vi "Deploy Firmware.vi"() -> ()   [LabVIEW 2011, in "LVH-LINX.lvlib"]
uses:
  LVH-LINX.lvlib
  Type Defs/Device Family.ctl
  Type Defs/Deploy Firmware State.ctl
panel:
  in  "Device Family Enum":T1
  out "Error Out":errorcluster
  in  "Error In":errorcluster
  out "Tab Control":T2(tab)
  in  "Device Help":bool
  in  "Firmware Program Interface":u16(ring) items=["Serial / USB"]
  in  "Device Type":u16(ring) items=["chipKIT Uno32", "chipKIT uC32", "chipKIT Max32", "chipKIT DP32"]
  in  "Device Family":u16(ring) items=["National Instruments", "Digilent", "Arduino"]
  in  "Device Cancel":bool
  in  "Device Next":bool
  in  "Int Help":bool
  in  "Int Previous":bool
  in  "Int Cancel":bool
  in  "Int Next":bool
  out "Interface Config":enum32{"N/A", "Serial / USB", "USB", "TCP"}(tab)
  in  "COM Port":refnum<visa-resource-name>
  in  "FWV Help":bool
  in  "FWV Cancel":bool
  in  "FWV Next":bool
  in  "FWV Previous":bool
  in  "Firmware Version":u16(ring)
  in  "Summary Next":bool
  in  "Summary Help":bool
  # "Choose The Device"
  # "!!! Could Add Test Connection Button Here !!!"
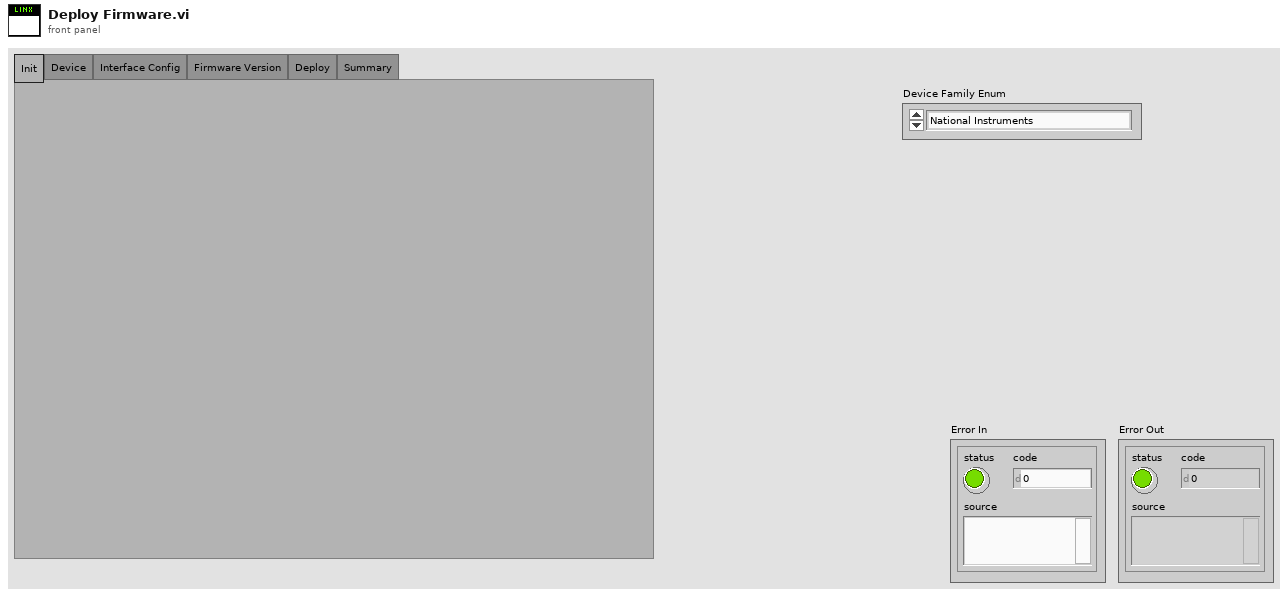
[diagram p1: front panel]
types:
  T1 = typedef "LVH-LINX.lvlib/Device Family.ctl" = enum8{"National Instruments", "Digilent", "Arduino"}
  T2 = enum32{"Init", "Device", "Interface Config", "Firmware Version", "Deploy", "Summary"}
  T3 = typedef "LVH-LINX.lvlib/Deploy Firmware State.ctl" = enum32{"Init", "Device", "Interface Config", "Firmware Version", "Deploy", "Summary"}
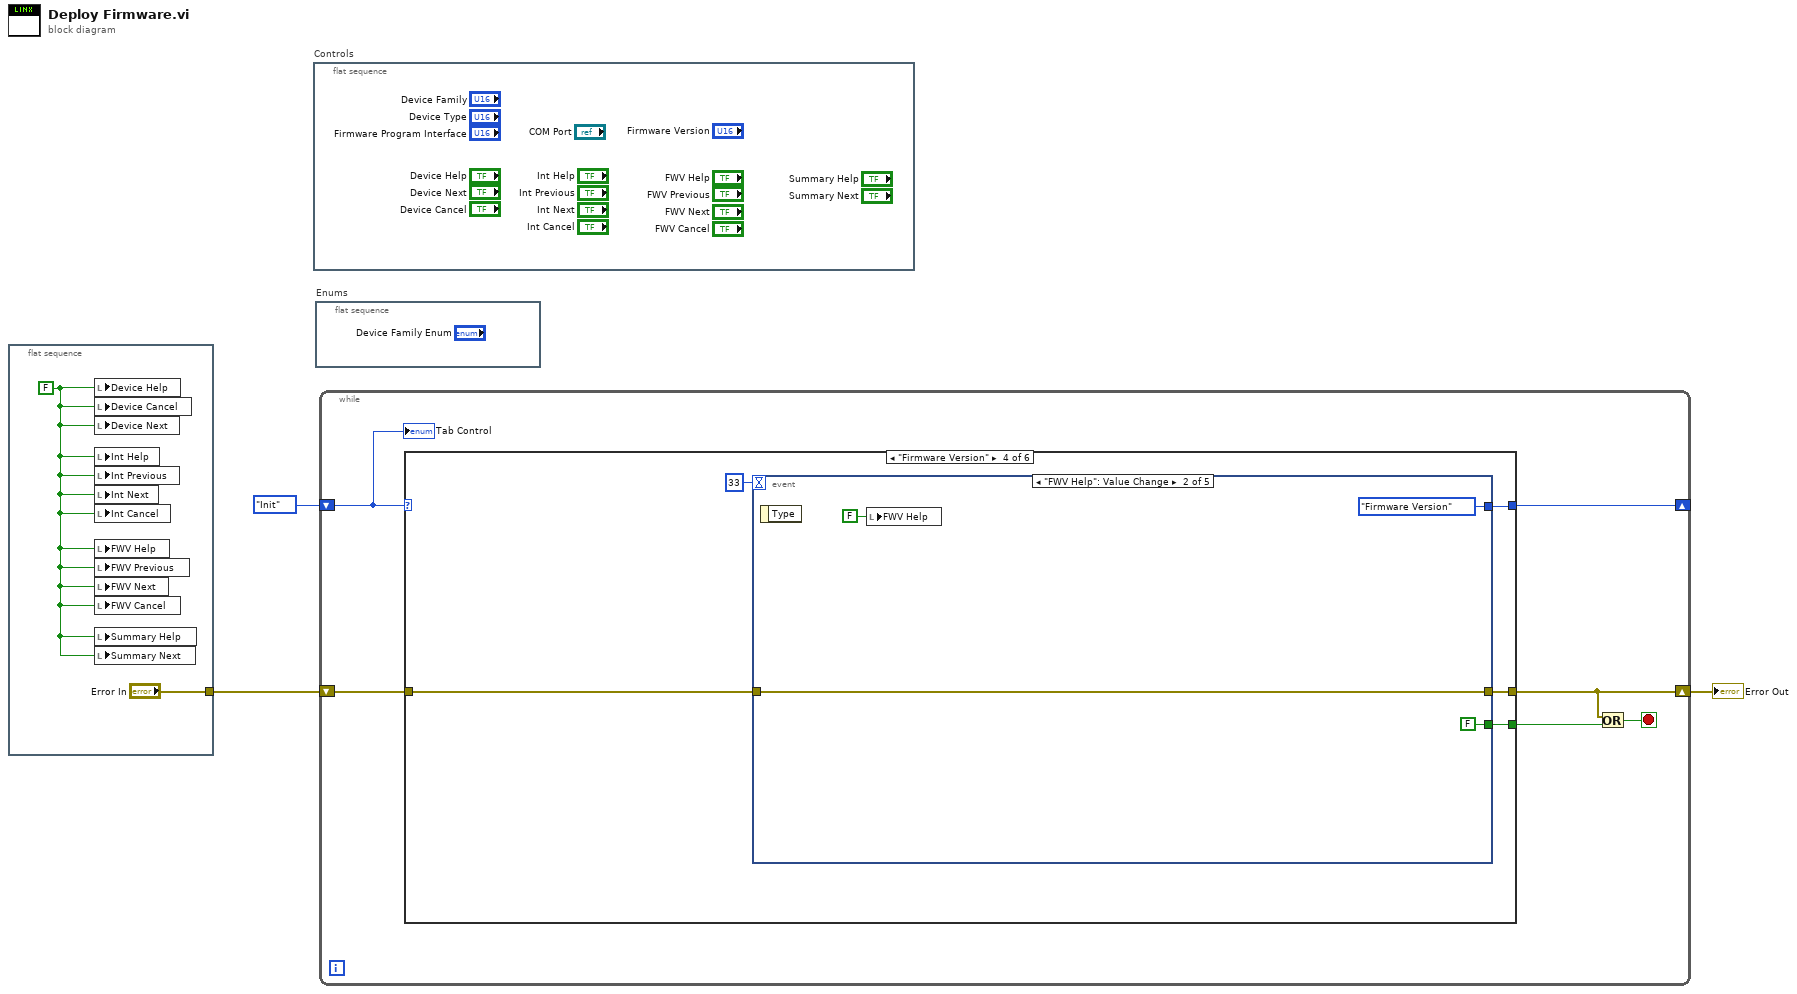
[diagram p0: block diagram]
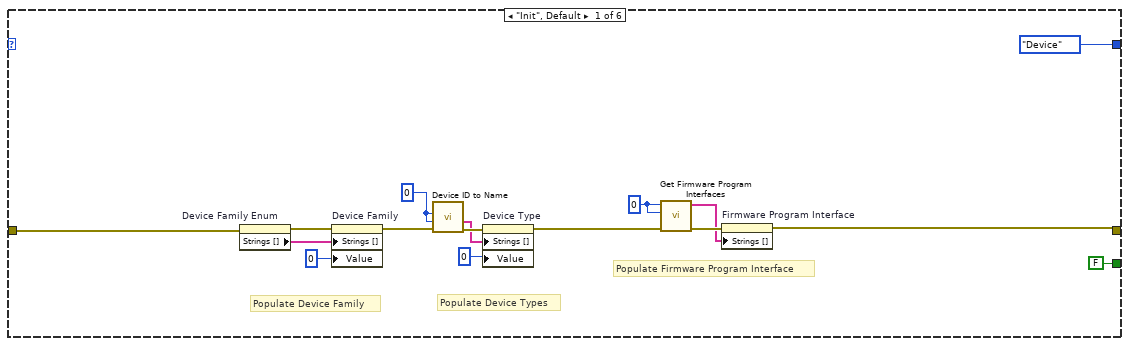
[diagram p2: hidden frame]
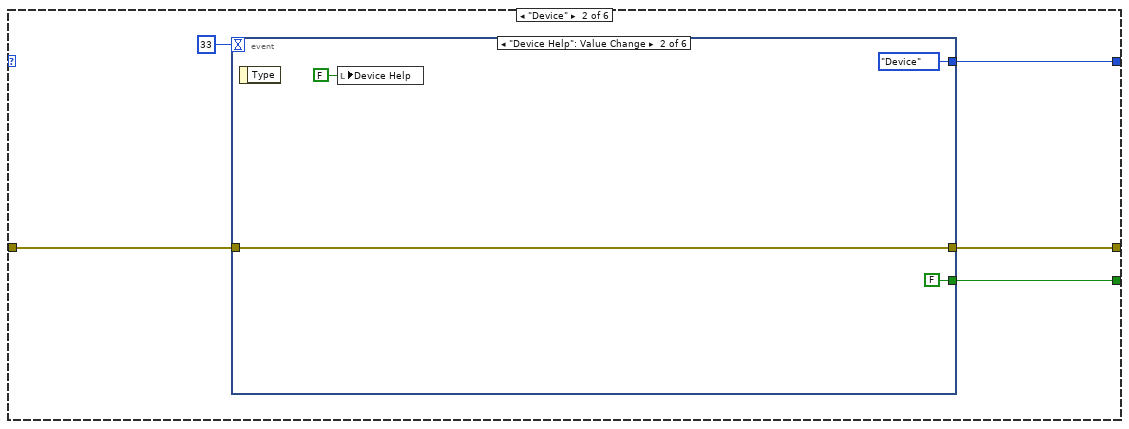
[diagram p3: hidden frame]
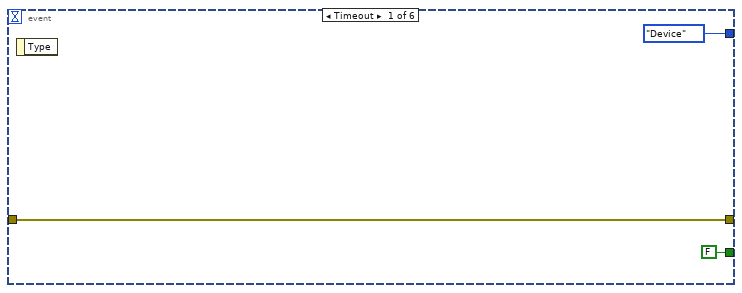
[diagram p4: hidden frame]
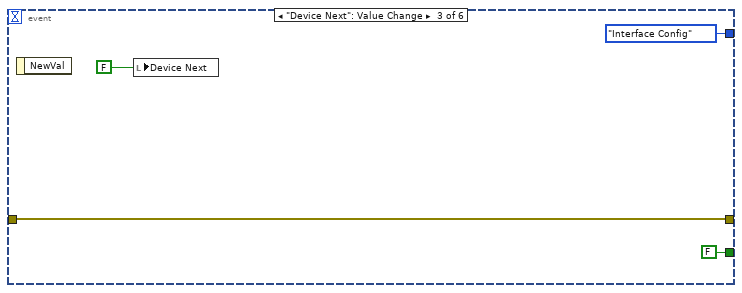
[diagram p5: hidden frame]
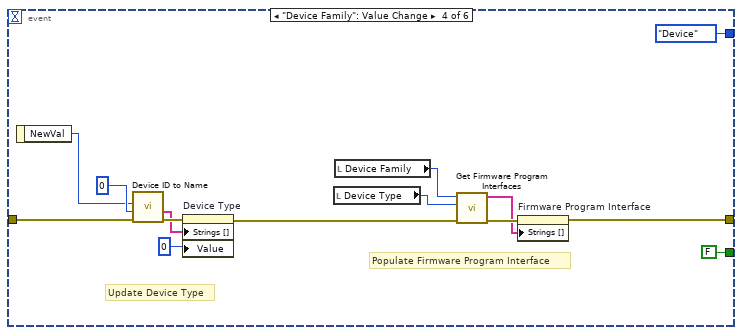
[diagram p6: hidden frame]
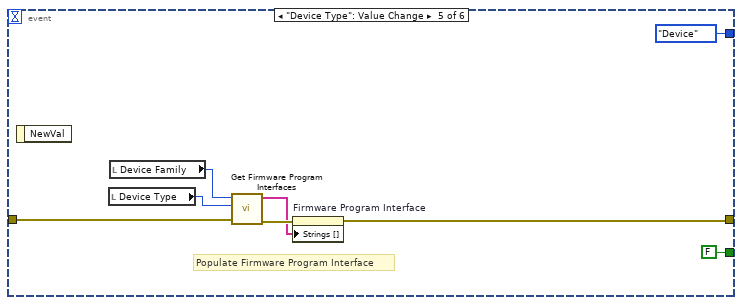
[diagram p7: hidden frame]
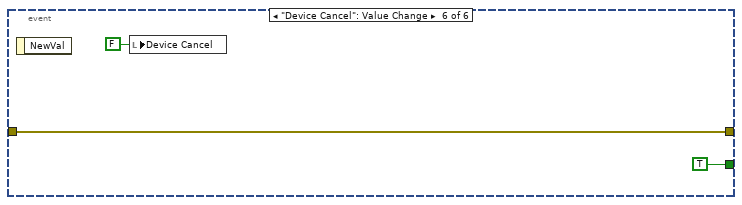
[diagram p8: hidden frame]
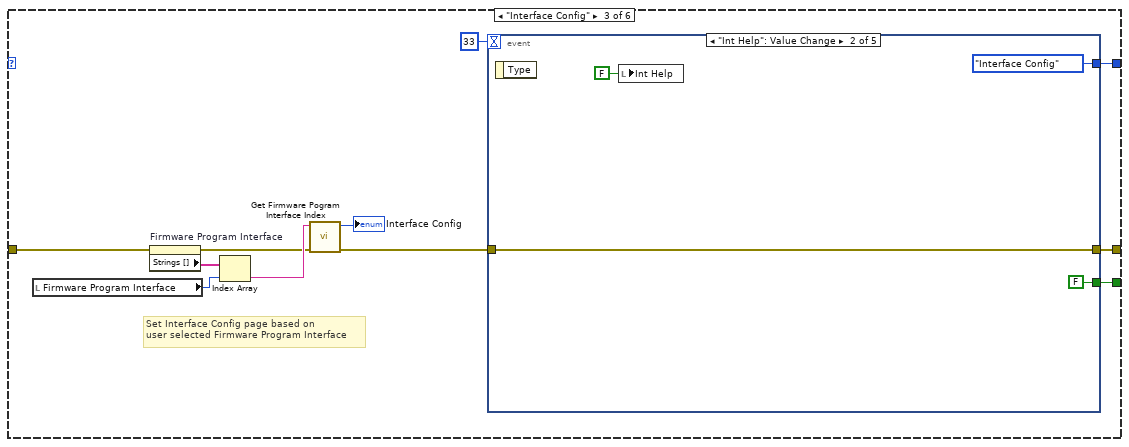
[diagram p9: hidden frame]
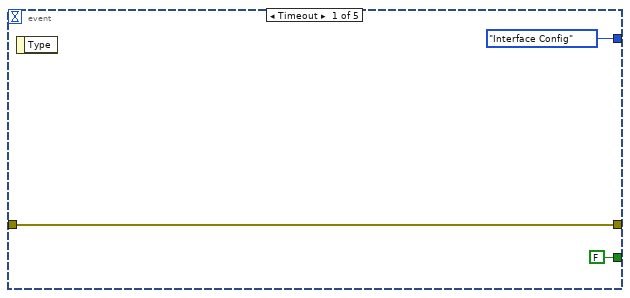
[diagram p10: hidden frame]
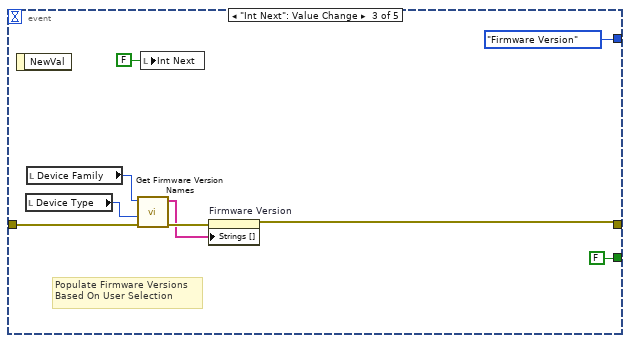
[diagram p11: hidden frame]
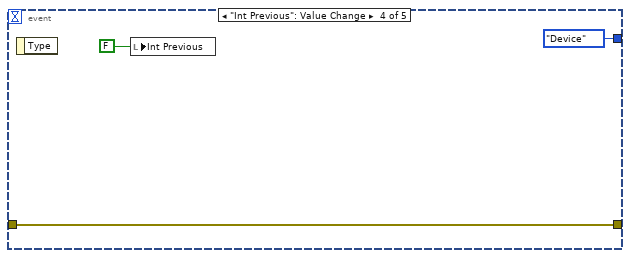
[diagram p12: hidden frame]
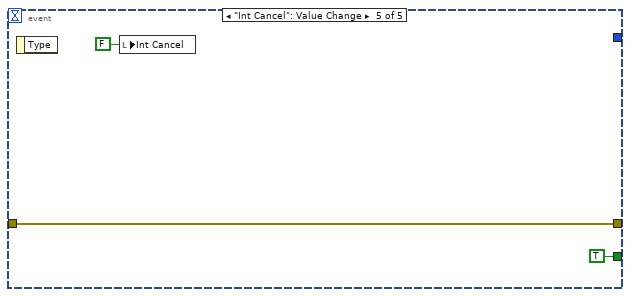
[diagram p13: hidden frame]
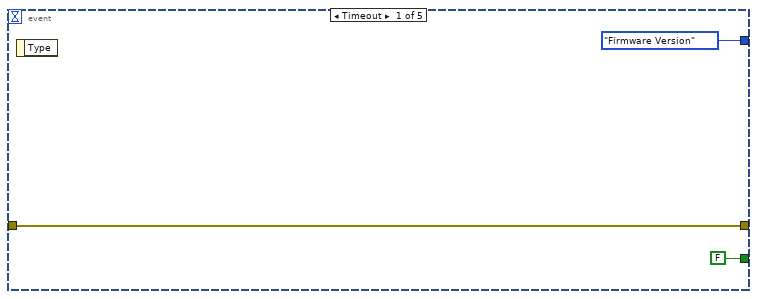
[diagram p14: hidden frame]
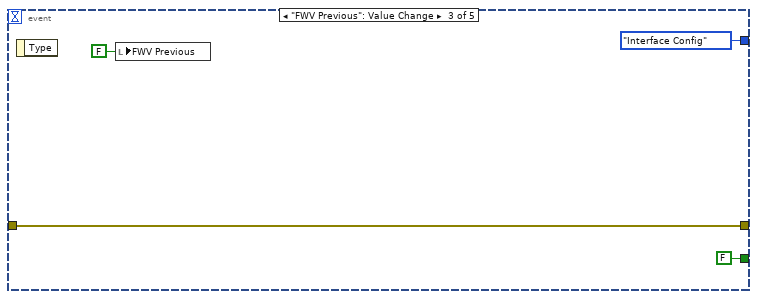
[diagram p15: hidden frame]
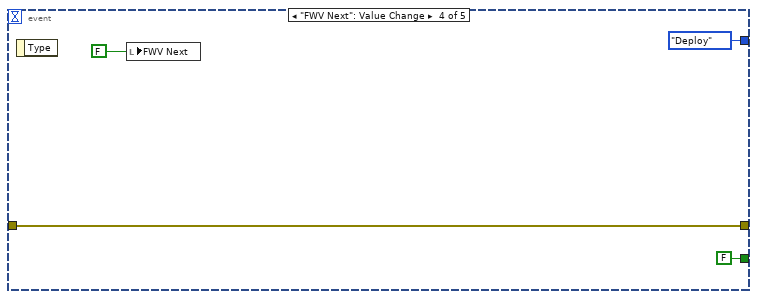
[diagram p16: hidden frame]
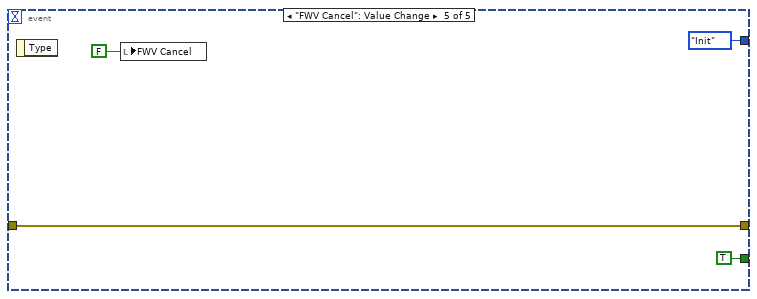
[diagram p17: hidden frame]
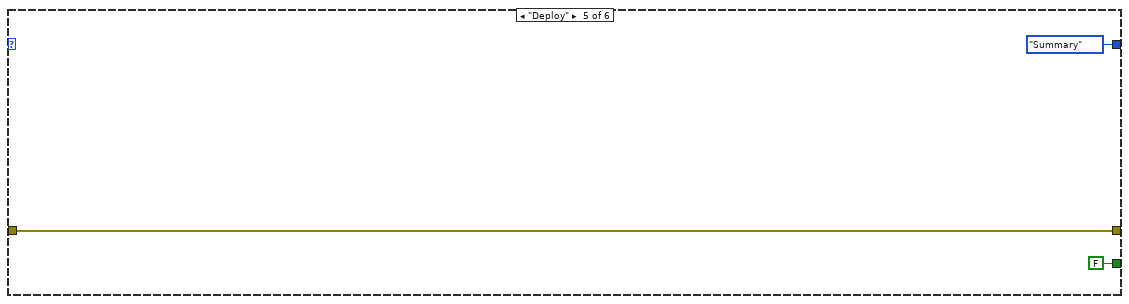
[diagram p18: hidden frame]
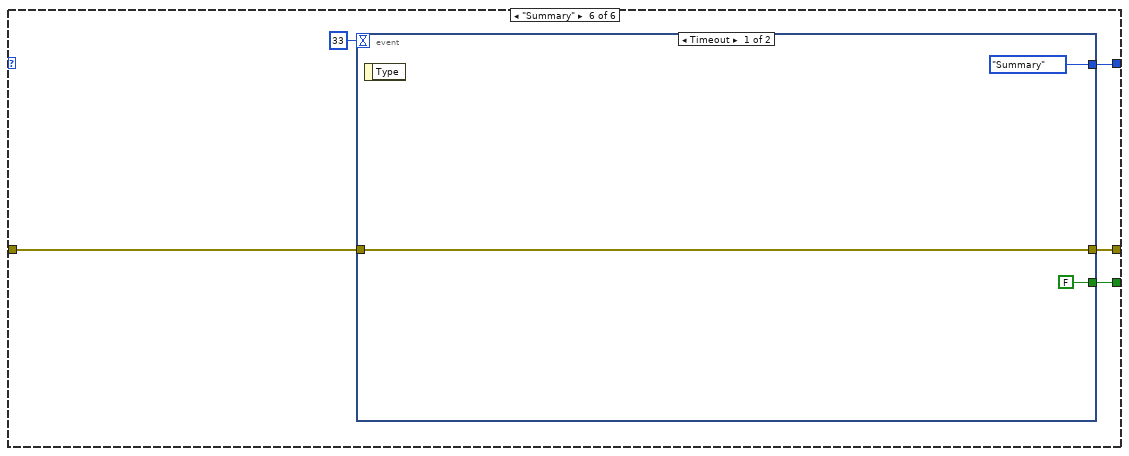
[diagram p19: hidden frame]
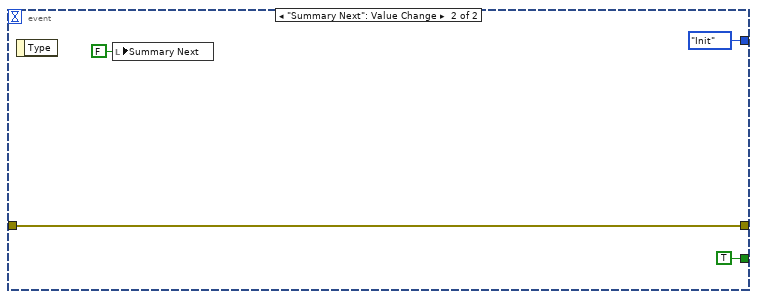
[diagram p20: hidden frame]
diagram:
  n1 = flat-sequence {
    tunnel: ["Error In"] -> w1
    frame #0 {
      w4 = FALSE ("Cancel")
      n2 = local write "Device Help"(w4) -> ()
      n3 = local write "Device Cancel"(w4) -> ()
      n4 = local write "Device Next"(w4) -> ()
      n5 = local write "Int Help"(w4) -> ()
      n6 = local write "Int Previous"(w4) -> ()
      n7 = local write "Int Next"(w4) -> ()
      n8 = local write "Int Cancel"(w4) -> ()
      n9 = local write "FWV Help"(w4) -> ()
      n10 = local write "FWV Previous"(w4) -> ()
      n11 = local write "FWV Next"(w4) -> ()
      n12 = local write "FWV Cancel"(w4) -> ()
      n13 = local write "Summary Help"(w4) -> ()
      n14 = local write "Summary Next"(w4) -> ()
    }
  }
  n15 = flat-sequence "Controls" {
    frame #0 {
    }
  }
  n16 = flat-sequence "Enums" {
    frame #0 {
    }
  }
  n17 = while {
    shift-right: [w9] -> _
    shift-left: Deploy_Firmware_State."Init" ("Deploy Firmware State") -> [w11]
    shift-right: [w8] -> w2
    shift-left: w1 -> [w10]
    stop <- w7 stop-if-true
    n18 = case shown="\"Firmware Version\"" w11 {
      tunnel: [w14 w31 w72 w106 w128 w133] -> w8
      tunnel: w10 -> [w13 w30 w78 w105 w128 w132]
      tunnel: [Deploy_Firmware_State."Device" ("Deploy Firmware State") w29 w79 w103 Deploy_Firmware_State."Summary" ("Deploy Firmware State") w130] -> w9
      tunnel: [FALSE w28 w69 w102 FALSE w129] -> w6
      frame "Init", Default {
        w15 = u32 0 ("Device Family")
        w21 = u32 0 ("Device Family")
        # "Populate Firmware Program Interface"
        # "Populate Device Types"
        # "Populate Device Family"
        n19 = property on="Device Family Enum" class="Enum (strict)"(error in=w13) -> (error out=w26:errorcluster, "Strings []"=w25:string[])  [unwired: 1 in, 1 out]
        n20 = property on="Device Family" class="Ring (strict)"(error in=w26, "Strings []"=w25, "Value"=u16 0 ("Device Family")) -> (error out=w23:errorcluster)  [unwired: 1 in, 1 out]
        n21 = call "Device ID to Name.vi"("Error In"=w23, "Device ID"=w21, "Device Family"=w21) -> ("Error Out"=w22:errorcluster, "Devices In Family"=w20:string[])  [unwired: 5 in, 2 out]
        n22 = property on="Device Type" class="Ring (strict)"(error in=w22, "Strings []"=w20, "Value"=u16 0 ("Device Family")) -> (error out=w16:errorcluster)  [unwired: 1 in, 1 out]
        n23 = call "Get Firmware Program Interfaces.vi"("Error In"=w16, "Device ID"=w15, "Device Family"=w15) -> ("Error Out"=w18:errorcluster, "Firmware Program Interfaces"=w17:string[])  [unwired: 7 in]
        n24 = property on="Firmware Program Interface" class="Ring (strict)"(error in=w18, "Strings []"=w17) -> (error out=w14:errorcluster)  [unwired: 1 in, 1 out]
      }
      frame "Device" {
        n25 = event shown="[1] \"Device Help\": Value Change" {
          selector: _ -> [_ _ _ _ _ _]
          dyn-events: _ -> [_ _ _ _ _ _]
          timeout: 33 -> [_ _ _ _ _ _]
          tunnel: [w35 w37 w42 w46 w62 w67] -> w31
          tunnel: w30 -> [w35 w37 w42 w53 w65 w67]
          tunnel: [Deploy_Firmware_State."Device" ("Deploy Firmware State") Deploy_Firmware_State."Device" ("Deploy Firmware State") Deploy_Firmware_State."Interface Config" ("Deploy Firmware State") Deploy_Firmware_State."Device" ("Deploy Firmware State") Deploy_Firmware_State."Device" ("Deploy Firmware State") _] -> w29
          tunnel: [FALSE FALSE FALSE FALSE FALSE TRUE] -> w28
          event Timeout {
            n26 = event-data() -> ()  [unwired: 1 in, 1 out]
          }
          event "Device Help": Value Change {
            n27 = event-data() -> ()  [unwired: 1 in, 1 out]
            n28 = local write "Device Help"(FALSE ("Device Help")) -> ()
          }
          event "Device Next": Value Change {
            n29 = event-data() -> ()  [unwired: 1 in, 1 out]
            n30 = local write "Device Next"(FALSE ("Next")) -> ()
          }
          event "Device Family": Value Change {
            # "Populate Firmware Program Interface"
            # "Update Device Type"
            n31 = event-data() -> ("NewVal"=w52:u16)  [unwired: 1 in]
            n32 = call "Device ID to Name.vi"("Error In"=w53, "Device ID"=u32 0 ("Device Family"), "Device Family"=w52) -> ("Error Out"=w57:errorcluster, "Devices In Family"=w55:string[])  [unwired: 5 in, 2 out]
            n33 = property on="Device Type" class="Ring (strict)"(error in=w57, "Strings []"=w55, "Value"=u16 0 ("Device Family")) -> (error out=w45:errorcluster)  [unwired: 1 in, 1 out]
            n34 = local read "Device Type"() -> (w48:u16)
            n35 = local read "Device Family"() -> (w47:u16)
            n36 = call "Get Firmware Program Interfaces.vi"("Error In"=w45, "Device ID"=w48, "Device Family"=w47) -> ("Error Out"=w50:errorcluster, "Firmware Program Interfaces"=w49:string[])  [unwired: 7 in]
            n37 = property on="Firmware Program Interface" class="Ring (strict)"(error in=w50, "Strings []"=w49) -> (error out=w46:errorcluster)  [unwired: 1 in, 1 out]
          }
          event "Device Type": Value Change {
            # "Populate Firmware Program Interface"
            n38 = event-data() -> ()  [unwired: 1 in, 1 out]
            n39 = local read "Device Type"() -> (w60:u16)
            n40 = local read "Device Family"() -> (w59:u16)
            n41 = call "Get Firmware Program Interfaces.vi"("Error In"=w65, "Device ID"=w60, "Device Family"=w59) -> ("Error Out"=w64:errorcluster, "Firmware Program Interfaces"=w63:string[])  [unwired: 7 in]
            n42 = property on="Firmware Program Interface" class="Ring (strict)"(error in=w64, "Strings []"=w63) -> (error out=w62:errorcluster)  [unwired: 1 in, 1 out]
          }
          event "Device Cancel": Value Change {
            n43 = event-data() -> ()  [unwired: 1 in, 1 out]
            n44 = local write "Device Cancel"(FALSE ("Device Cancel")) -> ()
          }
        }
      }
      frame "Interface Config" {
        # "Set Interface Config page based on \nuser selected Firmware Program Interface"
        n45 = local read "Firmware Program Interface"() -> (w76:u16)
        n46 = property on="Firmware Program Interface" class="Ring (strict)"(error in=w78) -> (error out=w74:errorcluster, "Strings []"=w77:string[])  [unwired: 1 in, 1 out]
        n47 = Index Array(array=w77, index=w76) -> (element=w75:string)
        n48 = call "Get Firmware Pogram Interface Index.vi"("Error In"=w74, "Firmware Program Interface"=w75) -> ("Error Out"=w71:errorcluster, "Interface Index"=→"Interface Config":i32)  [unwired: 8 in]
        n49 = event shown="[1] \"Int Help\": Value Change" {
          selector: _ -> [_ _ _ _ _]
          dyn-events: _ -> [_ _ _ _ _]
          timeout: 33 -> [_ _ _ _ _]
          tunnel: [Deploy_Firmware_State."Interface Config" ("Deploy Firmware State") Deploy_Firmware_State."Interface Config" ("Deploy Firmware State") Deploy_Firmware_State."Firmware Version" ("Deploy Firmware State") Deploy_Firmware_State."Device" ("Deploy Firmware State") _] -> w79
          tunnel: [w81 w86 w89 w98 w99] -> w72
          tunnel: w71 -> [w81 w86 w95 w98 w99]
          tunnel: [FALSE FALSE FALSE _ TRUE] -> w69
          event Timeout {
            n50 = event-data() -> ()  [unwired: 1 in, 1 out]
          }
          event "Int Help": Value Change {
            n51 = event-data() -> ()  [unwired: 1 in, 1 out]
            n52 = local write "Int Help"(FALSE ("Int Help")) -> ()
          }
          event "Int Next": Value Change {
            # "Populate Firmware Versions\nBased On User Selection"
            n53 = event-data() -> ()  [unwired: 1 in, 1 out]
            n54 = local read "Device Type"() -> (w92:u16)
            n55 = local read "Device Family"() -> (w91:u16)
            n56 = call "Get Firmware Version Names.vi"("Error In"=w95, "Device Family"=w92, "Device ID"=w91) -> ("Error Out"=w94:errorcluster, "Firmware Version Names"=w93:string[])  [unwired: 7 in]
            n57 = local write "Int Next"(FALSE ("Int Next")) -> ()
            n58 = property on="Firmware Version" class="Ring (strict)"(error in=w94, "Strings []"=w93) -> (error out=w89:errorcluster)  [unwired: 1 in, 1 out]
          }
          event "Int Previous": Value Change {
            n59 = event-data() -> ()  [unwired: 1 in, 1 out]
            n60 = local write "Int Previous"(FALSE ("Previous")) -> ()
          }
          event "Int Cancel": Value Change {
            n61 = event-data() -> ()  [unwired: 1 in, 1 out]
            n62 = local write "Int Cancel"(FALSE ("Int Cancel")) -> ()
          }
        }
      }
      frame "Firmware Version" {
        n63 = event shown="[1] \"FWV Help\": Value Change" {
          selector: _ -> [_ _ _ _ _]
          dyn-events: _ -> [_ _ _ _ _]
          timeout: 33 -> [_ _ _ _ _]
          tunnel: [w109 w113 w116 w120 w124] -> w106
          tunnel: w105 -> [w109 w113 w116 w120 w124]
          tunnel: [Deploy_Firmware_State."Firmware Version" ("Deploy Firmware State") Deploy_Firmware_State."Firmware Version" ("Deploy Firmware State") Deploy_Firmware_State."Interface Config" ("Deploy Firmware State") Deploy_Firmware_State."Deploy" ("Deploy Firmware State") Deploy_Firmware_State."Init" ("Deploy Firmware State")] -> w103
          tunnel: [FALSE FALSE FALSE FALSE TRUE] -> w102
          event Timeout {
            n64 = event-data() -> ()  [unwired: 1 in, 1 out]
          }
          event "FWV Help": Value Change {
            n65 = event-data() -> ()  [unwired: 1 in, 1 out]
            n66 = local write "FWV Help"(FALSE ("FWV Help")) -> ()
          }
          event "FWV Previous": Value Change {
            n67 = event-data() -> ()  [unwired: 1 in, 1 out]
            n68 = local write "FWV Previous"(FALSE ("FWV Previous")) -> ()
          }
          event "FWV Next": Value Change {
            n69 = event-data() -> ()  [unwired: 1 in, 1 out]
            n70 = local write "FWV Next"(FALSE ("FWV Previous")) -> ()
          }
          event "FWV Cancel": Value Change {
            n71 = event-data() -> ()  [unwired: 1 in, 1 out]
            n72 = local write "FWV Cancel"(FALSE ("FWV Previous")) -> ()
          }
        }
      }
      frame "Deploy" {
      }
      frame "Summary" {
        n73 = event shown="[0] Timeout" {
          selector: _ -> [_ _]
          dyn-events: _ -> [_ _]
          timeout: 33 -> [_ _]
          tunnel: [w136 w139] -> w133
          tunnel: w132 -> [w136 w139]
          tunnel: [Deploy_Firmware_State."Summary" ("Deploy Firmware State") Deploy_Firmware_State."Init" ("Deploy Firmware State")] -> w130
          tunnel: [FALSE TRUE] -> w129
          event Timeout {
            n74 = event-data() -> ()  [unwired: 1 in, 1 out]
          }
          event "Summary Next": Value Change {
            n75 = event-data() -> ()  [unwired: 1 in, 1 out]
            n76 = local write "Summary Next"(FALSE ("FWV Previous")) -> ()
          }
        }
      }
    }
    n77 = Or(x=w8, y=w6) -> (x .or. y?=w7:bool)
    "Tab Control" <- w11
  }
  "Error Out" <- w2
